vi "Atto DRY Interface get Magnetic Field.vi"(8 "error in (no error)":errorcluster, 11 "MagneticFieldT":sgl) -> (0 "error out":errorcluster, 2 "function return":i32, 3 "MagneticFieldT out":sgl)   [LabVIEW 2016, in "attoDRYLib.lvlib"]
doc: "int32_t __cdecl AttoDRY_Interface_getMagneticField(float *MagneticFieldT);"
uses:
  <userlib>/attoDRYLib/attoDRYLib.lvlib
  <userlib>/attoDRYLib/attoDRYLib.dll
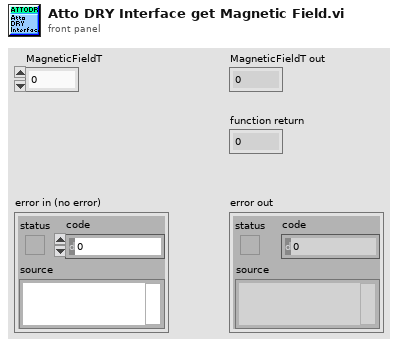
[diagram p1: front panel]
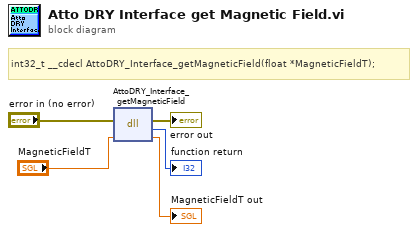
[diagram p0: block diagram]
diagram:
  # "int32_t __cdecl AttoDRY_Interface_getMagneticField(float *MagneticFieldT);"
  n1 = dll-call lib="C:/Program Files (x86)/National Instruments/LabVIEW 2016/user.lib/attoDRYLib/attoDRYLib.*" fn="AttoDRY_Interface_getMagneticField"(error in="error in (no error)", "MagneticFieldT"="MagneticFieldT") -> (error out=→"error out":errorcluster, →"function return":i32, "MagneticFieldT"=→"MagneticFieldT out":sgl)  [unwired: 2 in, 1 out]
